vi "MIC_Barcode read.vi"(8 "error in":errorcluster, 11 "queue in":refnum<queue>) -> (0 "error out":errorcluster, 1 "exit":bool, 2 "read buffer":string, 3 "queue Out 2":refnum<queue>)   [LabVIEW 2015]
uses:
  Test  enqueue/AutoTest seq.ctl
  <vilib>/Utility/error.llb/whitespace.ctl
  <vilib>/Instr/_visa.llb/VISA Configure Serial Port (Instr).vi
  Galobal variable_TI.vi
  Project Setup/Globle Variable/GR_Servo.vi
panel:
  out "x = y?":bool
  out "substring":string
  out "error out 2":errorcluster
  out "error out":errorcluster
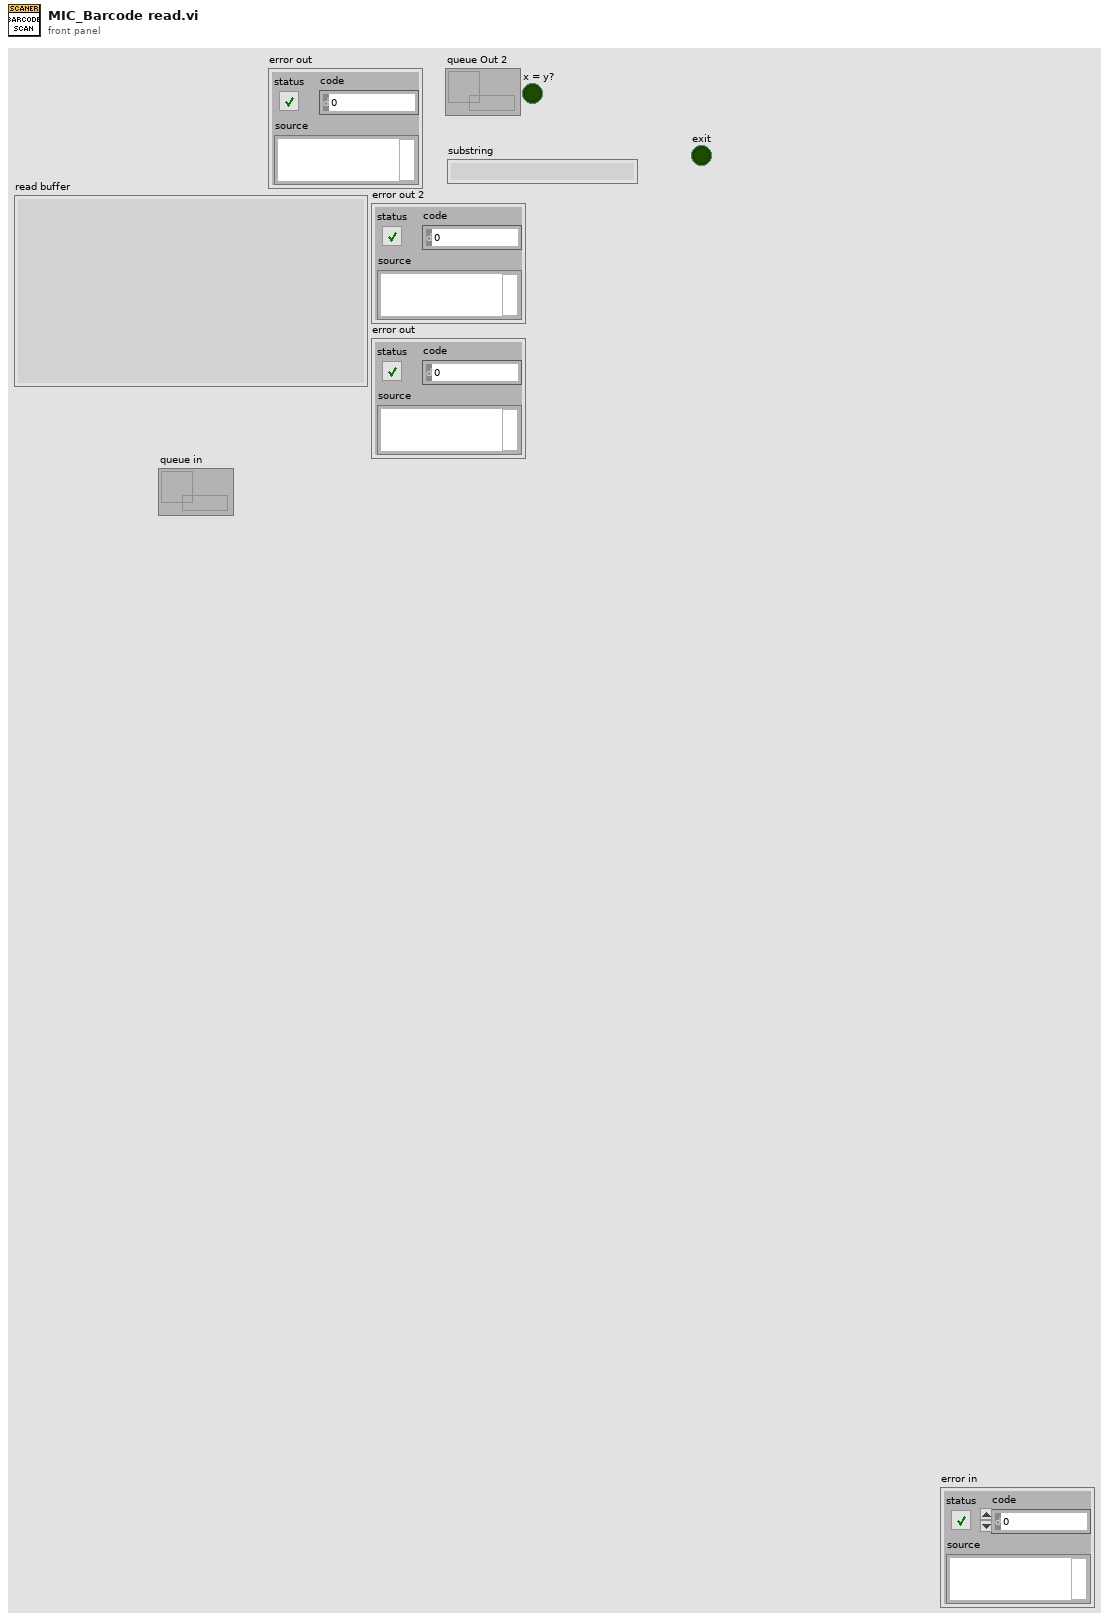
[diagram p1: front panel]
types:
  T1 = typedef "whitespace.ctl" = u16
  T2 = cluster{"MaxLoad(N) ":dbl, "Min Load(N)":dbl, "Load Offset":dbl, "Model":string, "MIC Code":string, "Dailcode1":string, "Dailcode2":string, "DailStrip1":string, "DailStrip2":string}
  T3 = cluster{"Start":bool, "Emergency ":bool, "Reset":bool, "Home":bool, "Safety":bool}
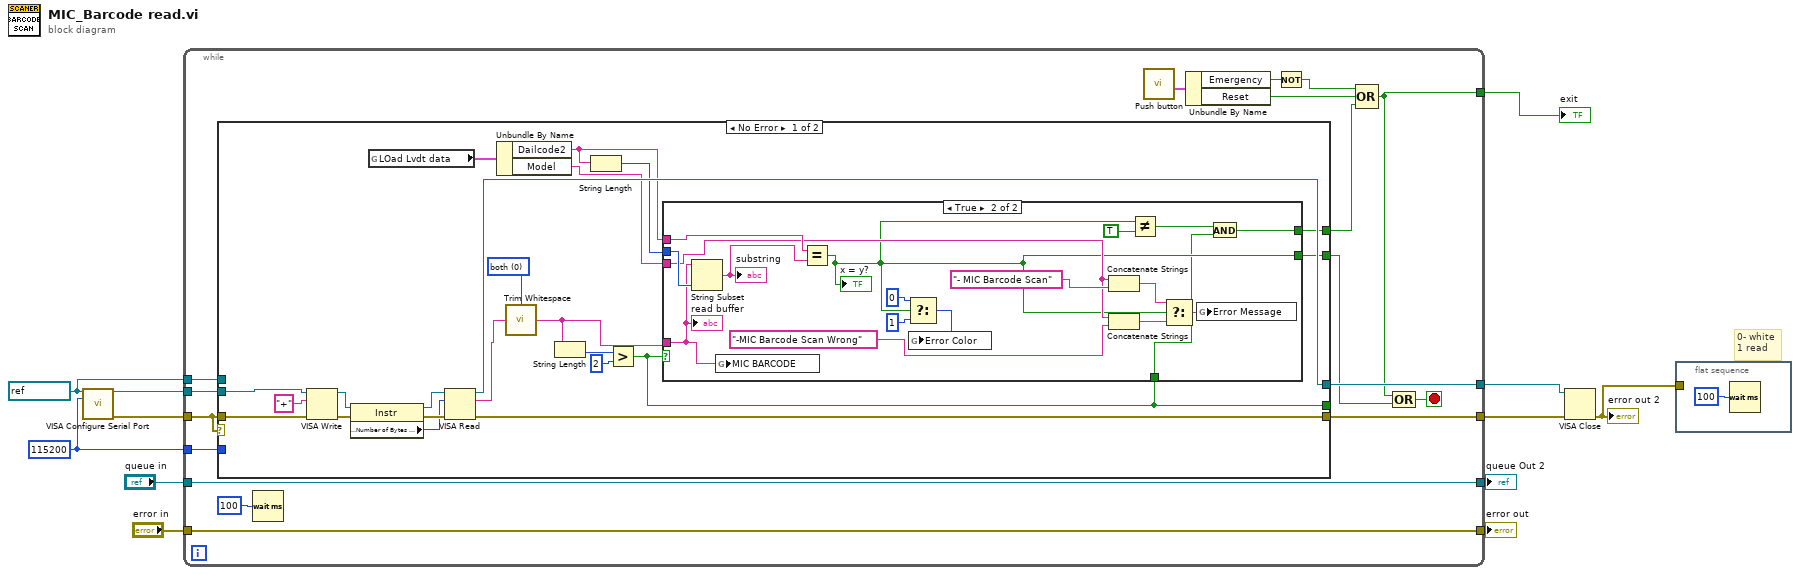
[diagram p0: block diagram]
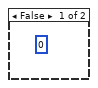
[diagram p2: hidden frame]
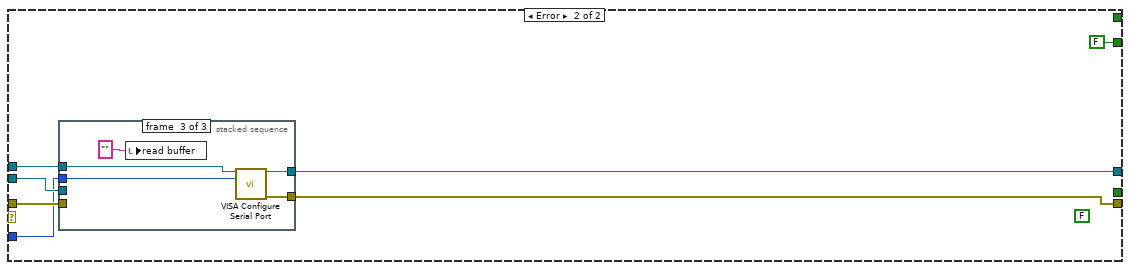
[diagram p3: hidden frame]
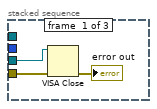
[diagram p4: hidden frame]
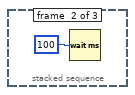
[diagram p5: hidden frame]
diagram:
  w7 = u32 115200 ("baud rate (9600)")
  w8 = refnum<visa-resource-name> "COM1" ("VISA resource name")
  # "0- white\n1 read"
  n1 = call-poly "VISA Configure Serial Port"("VISA resource name"=w8, "baud rate (9600)"=w7) -> ("VISA resource name out"=w12:refnum<visa-resource-name>, "error out"=w11:errorcluster)  [unwired: 12 in]
  n2 = while {
    tunnel: w12 -> [w29]
    tunnel: w11 -> [w27]
    tunnel: [w16] -> w10
    tunnel: [w28] -> w9
    tunnel: w8 -> [w26]
    tunnel: w7 -> [w25]
    tunnel: [w14] -> w6
    tunnel: [w22] -> w4
    tunnel: "queue in" -> [w22]
    tunnel: "error in" -> [w21]
    tunnel: [w21] -> w2
    stop <- w23 stop-if-true
    n3 = case shown="No Error" w27 {
      tunnel: w29 -> [w51 w76]
      tunnel: w27 -> [w50 w75]
      tunnel: [w49 w72] -> w16
      tunnel: [w48 w71] -> w28
      tunnel: w26 -> [_ w74]
      tunnel: w25 -> [_ w73]
      tunnel: [w36 FALSE] -> w15
      tunnel: [w31 _] -> _
      tunnel: [w30 _] -> w13
      frame No Error {
        w33 = T1 0 items=["both", "start of string", "end of string"] ("location (both)")
        n4 = VISA Write(VISA resource name=w51, write buffer="+", error in (no error)=w50) -> (VISA resource name out=w46:refnum<visa-resource-name>, error out=w47:errorcluster)  [unwired: 1 out]
        n5 = property class="Instr"(reference=w46, error in=w47) -> (reference out=w45:refnum<visa-resource-name>, error out=w44:errorcluster, "Serial Settings:Number of Bytes at Serial Port"=w43:u32)
        n6 = global read "Galobal variable_TI.vi" "LOad Lvdt data"() -> (w40:T2)
        n7 = VISA Read(VISA resource name=w45, byte count=w43, error in (no error)=w44) -> (VISA resource name out=w49:refnum<visa-resource-name>, read buffer=w34:string, error out=w48:errorcluster)  [unwired: 1 out]
        n8 = Unbundle By Name(w40) -> ("Dailcode2"=w39:string, "Model"=w37:string)
        n9 = call <vilib>:"Trim Whitespace.vi"("string"=w34, "location (both)"=w33) -> ("trimmed string"=w32:string)
        n10 = String Length(string=w32) -> (length=w42:i32)
        n11 = String Length(string=w39) -> (length=w38:i32)
        n12 = Greater?(x=w42, y=2) -> (0:w31:bool)
        n13 = case shown="True" w31 {
          tunnel: w32 -> [_ w57]
          tunnel: w39 -> [_ w68]
          tunnel: w38 -> [_ w69]
          tunnel: w37 -> [_ w59]
          tunnel: [_ w56] -> w36
          tunnel: w31 -> [_ w53]
          tunnel: [_ w52] -> w30
          frame False {
            (unwired) 0 ("f")
          }
          frame True {
            n14 = String Subset(string=w57, length (rest)=w69) -> (substring=w67:string)  [unwired: 1 in]
            "substring" <- w67
            n15 = global write "Galobal variable_TI.vi" "MIC BARCODE"(w57) -> ()
            n16 = Equal?(x=w68, y=w67) -> (x = y?=w56:bool)
            "x = y?" <- w56
            n17 = Select(t=0, s=w56, f=1) -> (s? t:f=w64:i32)
            n18 = global write "GR_Servo.vi" "Error Color"(w64) -> ()
            n19 = Concatenate Strings(w59, "- MIC Barcode Scan" ("string")) -> (w62:string)
            n20 = Concatenate Strings(w59, "-MIC Barcode Scan Wrong" ("string")) -> (w61:string)
            n21 = Not Equal?(x=w56, y=TRUE) -> (x != y?=w54:bool)
            n22 = Select(t=w62, s=w56, f=w61) -> (s? t:f=w60:string)
            n23 = global write "GR_Servo.vi" "Error Message"(w60) -> ()
            n24 = And(x=w54, y=w53) -> (x .and. y?=w52:bool)
            "read buffer" <- w57
          }
        }
      }
      frame Error {
        (unwired) FALSE
        n25 = stacked-sequence {
          tunnel: w76 -> [w78 _ _]
          tunnel: w75 -> [w77 _ _]
          tunnel: w74 -> [_ _ w85]
          tunnel: w73 -> [_ _ w84]
          tunnel: [_ _ w83] -> w72
          tunnel: [_ _ w82] -> w71
          frame #0 {
            n26 = VISA Close(VISA resource name=w78, error in (no error)=w77) -> (error out=→"error out":errorcluster)
          }
          frame #1 {
            n27 = Wait (ms)(milliseconds to wait=u32 100) -> ()  [unwired: 1 out]
          }
          frame #2 {
            n28 = local write "read buffer"("" ("read buffer")) -> ()
            n29 = call-poly "VISA Configure Serial Port"("VISA resource name"=w85, "baud rate (9600)"=w84) -> ("VISA resource name out"=w83:refnum<visa-resource-name>, "error out"=w82:errorcluster)  [unwired: 12 in]
          }
        }
      }
    }
    n30 = Wait (ms)(milliseconds to wait=u32 100) -> ()  [unwired: 1 out]
    n31 = call "Push button.vi"() -> ("Push Button"=w20:T3)  [unwired: 9 in, 2 out]
    n32 = Unbundle By Name(w20) -> ("Emergency"=w19:bool, "Reset"=w17:bool)
    n33 = Not(x=w19) -> (.not. x?=w18:bool)
    n34 = Compound Arithmetic op=OR(w18, w17, w13) -> (w14:bool)
    n35 = Compound Arithmetic op=OR(w14, w15) -> (w23:bool)
  }
  "exit" <- w6
  "queue Out 2" <- w4
  "error out" <- w2
  n36 = VISA Close(VISA resource name=w10, error in (no error)=w9) -> (error out=w1:errorcluster)
  "error out 2" <- w1
  n37 = flat-sequence {
    tunnel: w1 -> [_]
    frame #0 {
      n38 = Wait (ms)(milliseconds to wait=u32 100) -> ()  [unwired: 1 out]
    }
  }
